vi "Test.vi"() -> (0 "error out":errorcluster, 2 "ParsedData":T1)   [LabVIEW 2022 SP3]
uses:
  ArgumentParser/Source/ArgumentParser/_ParsedData.ctl
  ArgumentParser/Source/ArgumentParser/ArgumentParser.lvclass
  ArgumentParser/Source/ArgumentConfig/ArgumentConfig.lvclass
  ArgumentParser/Source/SubParserConfig/SubParserConfig.lvclass
  ArgumentParser/Source/ParserConfig/ParserConfig.lvclass
  ArgumentParser/Source/ArgumentParser/ArgumentParser.lvclass/ArgumentParser.ctl
  ArgumentParser/Source/SubParserConfig/SubParserConfig.lvclass/SubParserConfig.ctl
  ArgumentParser/Source/ParserConfig/ParserConfig.lvclass/ParserConfig.ctl
  ArgumentParser/Source/ArgumentConfig/ArgumentConfig.lvclass/ArgumentConfig.ctl
  ArgumentParser/Source/ParserConfig/Write Name.vi
  ArgumentParser/Source/ParserConfig/Write Aliases.vi
  ArgumentParser/Source/SubParserConfig/Write Title.vi
  ArgumentParser/Source/SubParserConfig/Write Description.vi
  ArgumentParser/Source/SubParserConfig/Write Destination.vi
  ArgumentParser/Source/SubParserConfig/Write Help.vi
  ArgumentParser/Source/ArgumentConfig/Write NameOrFlags.vi
  ArgumentParser/Source/ArgumentConfig/Write Help.vi
  ArgumentParser/Source/ArgumentParser/Write Program.vi
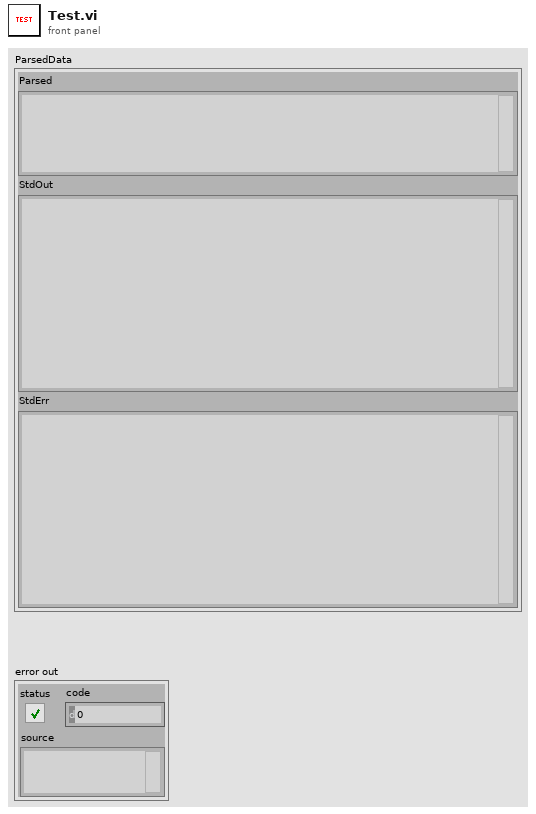
[diagram p1: front panel]
types:
  T1 = typedef "ArgumentParser.lvlib/ArgumentParser.lvclass/_ParsedData.ctl" = cluster{"Parsed":string, "StdOut":string, "StdErr":string}
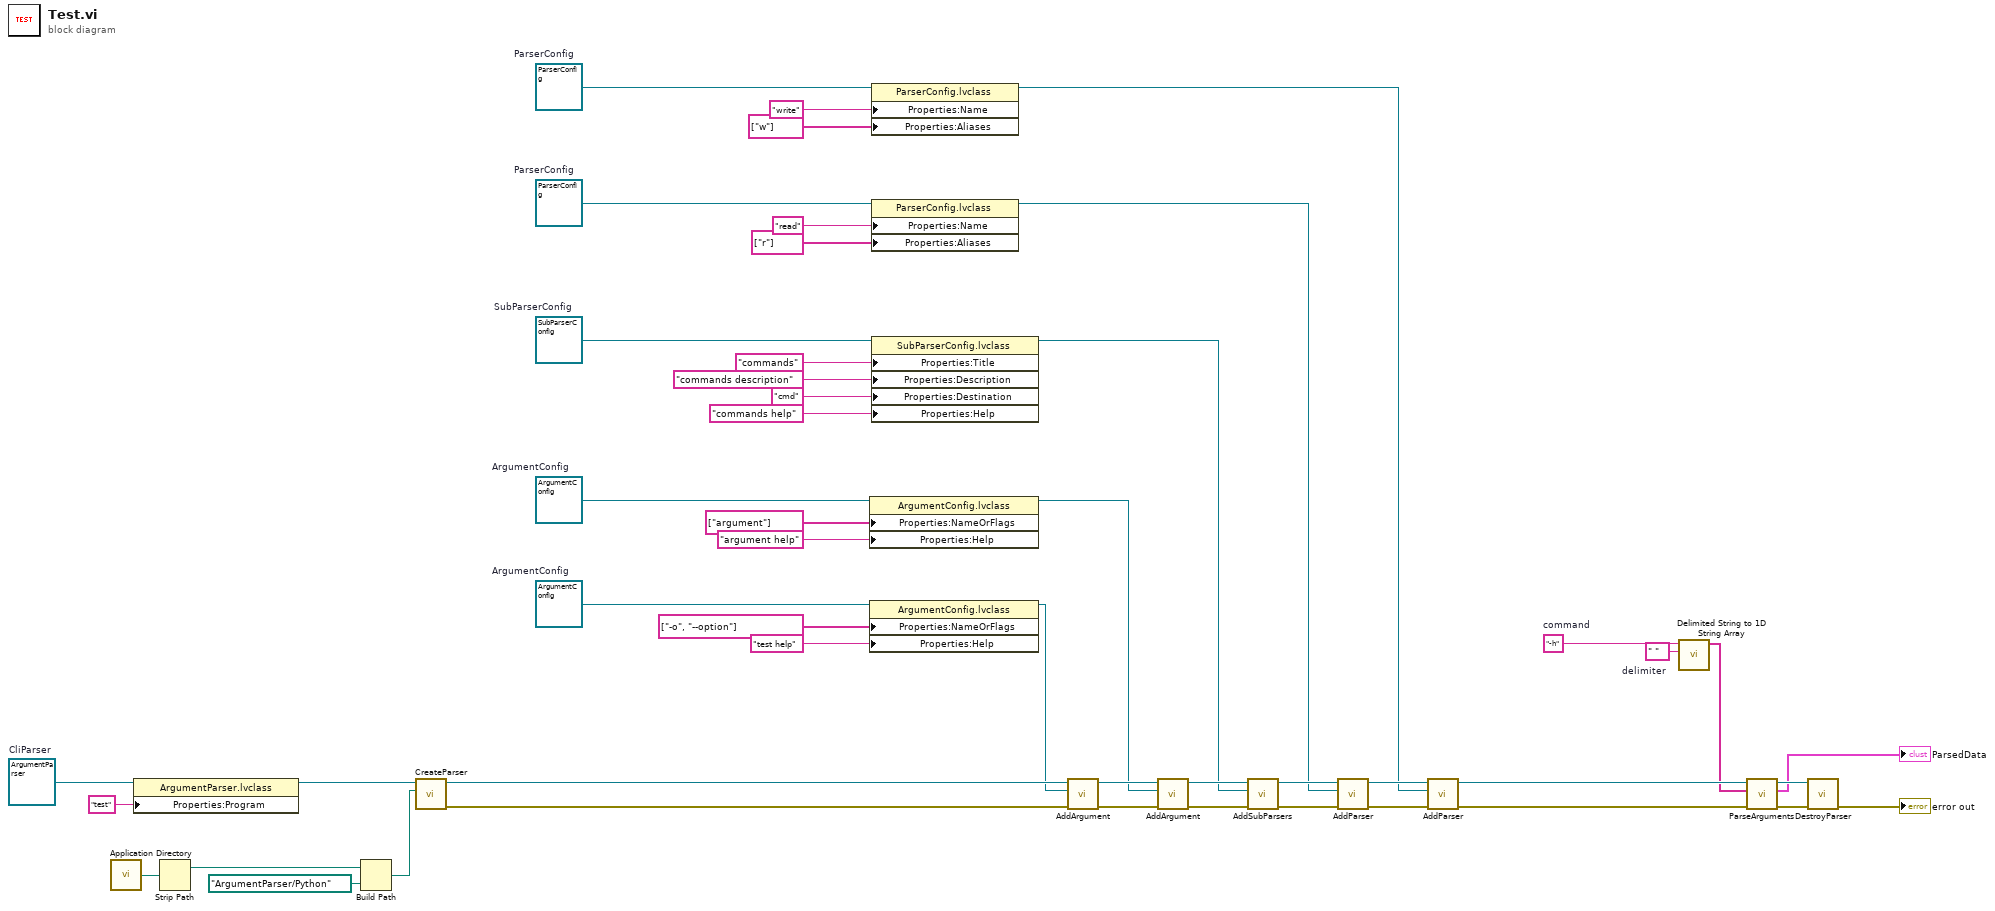
[diagram p0: block diagram]
diagram:
  w3 = " "  # delimiter
  w4 = "-h"  # command
  w9 = refnum<class "ParserConfig.lvclass"> refnum  # ParserConfig
  w15 = refnum<class "ParserConfig.lvclass"> refnum  # ParserConfig
  w23 = refnum<class "SubParserConfig.lvclass"> refnum  # SubParserConfig
  w31 = refnum<class "ArgumentConfig.lvclass"> refnum  # ArgumentConfig
  w42 = refnum<class "ArgumentConfig.lvclass"> refnum  # ArgumentConfig
  w48 = refnum<class "ArgumentParser.lvclass"> refnum  # CliParser
  n1 = call <vilib>:"Application Directory.vi"() -> ("Application Directory"=w46:path)
  n2 = property class="ArgumentParser.lvclass"(reference=w48, "Properties:Program"="test" ("Program")) -> (reference out=w27:refnum<class "ArgumentParser.lvclass">)  [unwired: 1 in, 1 out]
  n3 = Strip Path(path=w46) -> (stripped path=w1:path)  [unwired: 1 out]
  n4 = Build Path(base path=w1, name or relative path=path "ArgumentParser/Python") -> (appended path=w45:path)
  n5 = call-dynamic "CreateParser.vi"("PythonModuleDirectory"=w45, "ArgumentParser in"=w27) -> ("error out"=w43:errorcluster, "ArgumentParser out"=w44:refnum<class "ArgumentParser.lvclass">)  [unwired: 8 in]
  n6 = property class="ArgumentConfig.lvclass"(reference=w31, "Properties:NameOrFlags"=string[] ["argument"] ("NameOrFlags"), "Properties:Help"="argument help" ("Help")) -> (reference out=w28:refnum<class "ArgumentConfig.lvclass">)  [unwired: 1 in, 1 out]
  n7 = property class="ArgumentConfig.lvclass"(reference=w42, "Properties:NameOrFlags"=string[] ["-o", "--option"] ("NameOrFlags"), "Properties:Help"="test help" ("Help")) -> (reference out=w41:refnum<class "ArgumentConfig.lvclass">)  [unwired: 1 in, 1 out]
  n8 = property class="ParserConfig.lvclass"(reference=w9, "Properties:Name"="write" ("Name"), "Properties:Aliases"=string[] ["w"] ("Aliases")) -> (reference out=w5:refnum<class "ParserConfig.lvclass">)  [unwired: 1 in, 1 out]
  n9 = property class="ParserConfig.lvclass"(reference=w15, "Properties:Name"="read" ("Name"), "Properties:Aliases"=string[] ["r"] ("Aliases")) -> (reference out=w14:refnum<class "ParserConfig.lvclass">)  [unwired: 1 in, 1 out]
  n10 = property class="SubParserConfig.lvclass"(reference=w23, "Properties:Title"="commands" ("Title"), "Properties:Description"="commands description" ("Description"), "Properties:Destination"="cmd" ("Destination"), "Properties:Help"="commands help" ("Help")) -> (reference out=w22:refnum<class "SubParserConfig.lvclass">)  [unwired: 1 in, 1 out]
  n11 = call-dynamic "AddArgument.vi"("error in (no error)"=w43, "ArgumentConfig"=w41, "ArgumentParser in"=w44) -> ("error out"=w38:errorcluster, "ArgumentParser out"=w29:refnum<class "ArgumentParser.lvclass">)  [unwired: 7 in]
  n12 = call-dynamic "AddArgument.vi"("error in (no error)"=w38, "ArgumentConfig"=w28, "ArgumentParser in"=w29) -> ("error out"=w30:errorcluster, "ArgumentParser out"=w24:refnum<class "ArgumentParser.lvclass">)  [unwired: 7 in]
  n13 = call-dynamic "AddSubParsers.vi"("error in (no error)"=w30, "SubParserConfig"=w22, "ArgumentParser in"=w24) -> ("error out"=w25:errorcluster, "ArgumentParser out"=w16:refnum<class "ArgumentParser.lvclass">)  [unwired: 7 in]
  n14 = call-dynamic "AddParser.vi"("error in (no error)"=w25, "ParserConfig"=w14, "ArgumentParser in"=w16) -> ("error out"=w17:errorcluster, "ArgumentParser out"=w7:refnum<class "ArgumentParser.lvclass">)  [unwired: 7 in]
  n15 = call-dynamic "AddParser.vi"("error in (no error)"=w17, "ParserConfig"=w5, "ArgumentParser in"=w7) -> ("error out"=w8:errorcluster, "ArgumentParser out"=w6:refnum<class "ArgumentParser.lvclass">)  [unwired: 7 in]
  n16 = call <vilib>:"Delimited String to 1D String Array.vi"("delimiter"=w3, "delimited string"=w4) -> ("string array"=w2:string[])  [unwired: 9 in]
  n17 = call-dynamic "ParseArguments.vi"("error in (no error)"=w8, "CliArguments"=w2, "ArgumentParser in"=w6) -> ("error out"=w36:errorcluster, "ParsedData"=→"ParsedData":T1, "ArgumentParser out"=w37:refnum<class "ArgumentParser.lvclass">)  [unwired: 6 in]
  n18 = call-dynamic "DestroyParser.vi"("error in (no error)"=w36, "ArgumentParser in"=w37) -> ("error out"=→"error out":errorcluster)  [unwired: 8 in, 1 out]
